vi "Version_2.0_Single_Column_Code.vi"() -> ()   [LabVIEW 2020] (continued)
                          }
                          frame #3 {
                            n8961 = local read "Stopper that ends \nthe main loops"() -> (w9454:bool)
                            n8962 = local read "VISA Refnum in\nfor Pump"() -> (w9455:refnum<visa-resource-name>)
                            n8963 = case shown="True" w9454 {
                              frame False {
                              }
                              frame True {
                                n8964 = local read "VISA Refnum in\nfor Pump"() -> (w9456:refnum<visa-resource-name>)
                                n8965 = call "HardStopCurrentProcess (SubVI).vi"("VISA Refnum in"=w9456) -> ()  [unwired: 11 in]
                              }
                            }
                            n8966 = call "ProcessCompletionWaiter (SubVI).vi"("VISA Refnum in"=w9455) -> ()  [unwired: 11 in]
                          }
                          frame #4 {
                            # "Reads the initial Plunger Position for computing the volume dispensed"
                            n8967 = local read "VISA Refnum in\nfor Pump"() -> (w9458:refnum<visa-resource-name>)
                            n8968 = call "AbsolutePlungerPosition (SubVI).vi"("VISA Refnum in"=w9458) -> ("Plunger Position"=w9457:i32)  [unwired: 10 in]
                            n8969 = local write "Initial Plunger Position"(w9457) -> ()
                          }
                          frame #5 {
                            # "Switch to Port-10"
                            # "Port-10 of the pump is conncted to column-2 of chip"
                            n8970 = local read "VISA Refnum in\nfor Pump"() -> (w9460:refnum<visa-resource-name>)
                            n8971 = call "PortChanger (SubVI).vi"("Port Number"="10", "VISA Refnum in"=w9460) -> ()  [unwired: 10 in]
                          }
                          frame #6 {
                            n8972 = local read "Stopper that ends \nthe main loops"() -> (w9461:bool)
                            n8973 = local read "VISA Refnum in\nfor Pump"() -> (w9462:refnum<visa-resource-name>)
                            n8974 = case shown="True" w9461 {
                              frame False {
                              }
                              frame True {
                                n8975 = local read "VISA Refnum in\nfor Pump"() -> (w9463:refnum<visa-resource-name>)
                                n8976 = call "HardStopCurrentProcess (SubVI).vi"("VISA Refnum in"=w9463) -> ()  [unwired: 11 in]
                              }
                            }
                            n8977 = call "ProcessCompletionWaiter (SubVI).vi"("VISA Refnum in"=w9462) -> ()  [unwired: 11 in]
                          }
                          frame #7 {
                            # "Keeps the AMF valve after column-1 closed and valve after column-2 open"
                            n8978 = local read "Buffer-C2 Dispense\nFlow Rate (ul/min)"() -> (w9476:dbl)
                            n8979 = local read "Buffer-C2 Pumping\nResolution"() -> (w9475:T2)
                            n8980 = local read "VISA Refnum in\nfor Pump"() -> (w9478:refnum<visa-resource-name>)
                            n8981 = local write "Pause Data Collection"(FALSE ("Pause Data Collection")) -> ()
                            n8982 = local write "Valve V1 Open"(FALSE ("Valve V1 Open")) -> ()
                            n8983 = local write "Valve V3 Open"(TRUE ("Valve V3 Open")) -> ()
                            n8984 = local write "Valve V2 Open"(FALSE ("Valve V2 Open")) -> ()
                            n8985 = local write "Valve V4 Open"(TRUE ("Valve V4 Open")) -> ()
                            n8986 = local read "Volume of Syringe"() -> (w9477:dbl)
                            n8987 = call "GoToAbsolutePosition(SubVI).vi"("Absolute Volume Position in Syringe (in ul)"=0.0 ("Volume to be Dispensed"), "Volume of Syringe"=w9477, "Resolution of Pumping"=w9475, "Flow Rate (ul/min)"=w9476, "VISA Refnum in"=w9478) -> ()  [unwired: 6 in, 1 out]
                            n8988 = local write "External Valve \nOpen"(FALSE ("External Valve \nOpen")) -> ()
                            n8989 = local write "Valve V8 Open"(FALSE ("Valve V8 Open")) -> ()
                            n8990 = local write "Valve V7 Open"(TRUE ("Valve V7 Open")) -> ()
                            n8991 = local write "Valve V6 Open"(TRUE ("Valve V6 Open")) -> ()
                            n8992 = local write "Valve V5 Open"(TRUE ("Valve V5 Open")) -> ()
                          }
                          frame #8 {
                            n8993 = local read "Initial Plunger Position"() -> (w9481:dbl)
                            n8994 = local read "Buffer-C2 Pumping\nResolution"() -> (w9480:T2)
                            n8995 = local read "VISA Refnum in\nfor Pump"() -> (w9482:refnum<visa-resource-name>)
                            n8996 = local read "Volume of Syringe"() -> (w9479:dbl)
                            n8997 = while {
                              tunnel: w9481 -> [w9488]
                              tunnel: w9482 -> [w9487]
                              tunnel: w9480 -> [w9486]
                              tunnel: w9479 -> [w9485]
                              stop <- w9483 stop-if-true
                              n8998 = Wait (ms)(milliseconds to wait=u32 100) -> ()  [unwired: 1 out]
                              n8999 = stacked-sequence {
                                tunnel: w9488 -> [w9494 _]
                                tunnel: w9487 -> [w9493 w9514]
                                tunnel: w9486 -> [w9492 _]
                                tunnel: w9485 -> [w9491 _]
                                tunnel: [_ w9511] -> w9483
                                frame #0 {
                                n9000 = call "AbsolutePlungerPosition (SubVI).vi"("VISA Refnum in"=w9493) -> ("Plunger Position"=w9490:i32)  [unwired: 10 in]
                                n9001 = case shown="\"Standard Pumping\", Default" w9492 {
                                tunnel: w9494 -> [w9499 w9508]
                                tunnel: w9490 -> [w9500 w9507]
                                tunnel: [w9498 w9505] -> w9489
                                tunnel: w9491 -> [w9497 w9506]
                                frame "Standard Pumping", Default {
                                n9002 = Subtract(x=w9499, y=w9500) -> (x-y=w9496:dbl)
                                n9003 = Absolute Value(x=w9496) -> (abs(x)=w9495:dbl)
                                n9004 = Multiply(x=w9495, y=w9497) -> (x*y=w9502:dbl)
                                n9005 = Divide(x=w9502, y=3000.0) -> (x/y=w9498:dbl)
                                }
                                frame "High Resolution Pumping" {
                                n9006 = Subtract(x=w9508, y=w9507) -> (x-y=w9504:dbl)
                                n9007 = Absolute Value(x=w9504) -> (abs(x)=w9503:dbl)
                                n9008 = Multiply(x=w9503, y=w9506) -> (x*y=w9510:dbl)
                                n9009 = Divide(x=w9510, y=24000.0) -> (x/y=w9505:dbl)
                                }
                                }
                                n9010 = local write "Volume being Injected \nin this process"(w9489) -> ()
                                }
                                frame #1 {
                                n9011 = call "LSPOneStatus (SubVI).vi"("VISA Refnum in"=w9514) -> ("read buffer"=w9516:string)  [unwired: 10 in]
                                n9012 = local read "Stopper that ends \nthe main loops"() -> (w9513:bool)
                                n9013 = call <vilib>:"Trim Whitespace.vi"("string"=w9516) -> ("trimmed string"=w9515:string)  [unwired: 1 in]
                                n9014 = Equal?(x=w9515, y="/0`\u0003") -> (x = y?=w9512:bool)
                                n9015 = Or(x=w9512, y=w9513) -> (x .or. y?=w9511:bool)
                                }
                              }
                            }
                          }
                          frame #9 {
                            n9016 = local read "Stop for End of \nExperiment \nand Data Writing"() -> (w9518:bool)
                            n9017 = local write "Pause Data Collection"(TRUE ("Pause Data Collection")) -> ()
                            n9018 = local write "Valve V2 Open"(FALSE ("Valve V2 Open")) -> ()
                            n9019 = local write "Valve V1 Open"(FALSE ("Valve V1 Open")) -> ()
                            n9020 = local write "Valve V3 Open"(FALSE ("Valve V3 Open")) -> ()
                            n9021 = local write "Valve V4 Open"(FALSE ("Valve V4 Open")) -> ()
                            n9022 = local write "Start the Process"(FALSE) -> ()
                            n9023 = Wait (ms)(milliseconds to wait=u32 500) -> ()  [unwired: 1 out]
                            n9024 = case shown="True" w9518 {
                              frame False {
                              }
                              frame True {
                                n9025 = local read "VISA Refnum in\nfor Pump"() -> (w9531:refnum<visa-resource-name>)
                                n9026 = call "HardStopCurrentProcess (SubVI).vi"("VISA Refnum in"=w9531) -> ()  [unwired: 11 in]
                              }
                            }
                            n9027 = local write "External Valve \nOpen"(FALSE ("External Valve \nOpen")) -> ()
                            n9028 = local write "Valve V8 Open"(FALSE ("Valve V8 Open")) -> ()
                            n9029 = local write "Valve V6 Open"(FALSE ("Valve V6 Open")) -> ()
                            n9030 = local write "Valve V5 Open"(FALSE ("Valve V5 Open")) -> ()
                            n9031 = local write "Valve V7 Open"(FALSE ("Valve V7 Open")) -> ()
                          }
                          frame #10 {
                            n9032 = local write "Volume being Injected \nin this process"(0.0 ("Volume being Injected \nin this process")) -> ()
                          }
                        }
                      }
                    }
                  }
                }
              }
              frame True {
                n9033 = local write "Pause Data Collection"(FALSE ("Pause Data Collection")) -> ()
              }
            }
          }
          frame "Initialize Only the Valve" {
            n9034 = local read "Stop for End of \nExperiment \nand Data Writing"() -> (w9534:bool)
            n9035 = case shown="False" w9534 {
              frame False {
                n9036 = local read "Start the Process"() -> (w9535:bool)
                n9037 = case shown="True" w9535 {
                  frame False {
                    n9038 = local read "Stopper that ends \nthe main loops"() -> (w9537:bool)
                    n9039 = local read "Start the Process"() -> (w9538:bool)
                    n9040 = Or(x=w9538, y=w9537) -> (x .or. y?=w9536:bool)
                    n9041 = case shown="False" w9536 {
                      frame False {
                        n9042 = while {
                          stop <- w9541 stop-if-true
                          n9043 = local read "Stopper that ends \nthe main loops"() -> (w9543:bool)
                          n9044 = local read "Start the Process"() -> (w9542:bool)
                          n9045 = Or(x=w9542, y=w9543) -> (x .or. y?=w9541:bool)
                          n9046 = Wait (ms)(milliseconds to wait=u32 10) -> ()  [unwired: 1 out]
                        }
                        n9047 = One Button Dialog(message="Please select the process and press the 'Start Process' Button") -> ()  [unwired: 1 in, 1 out]
                      }
                      frame True {
                      }
                    }
                  }
                  frame True {
                    n9048 = stacked-sequence {
                      frame #0 {
                        n9049 = local read "VISA Refnum in\nfor Valve"() -> (w9544:refnum<visa-resource-name>)
                        n9050 = call "Initializer_Valve (SubVI).vi"("VISA Refnum in"=w9544) -> ()  [unwired: 11 in]
                      }
                      frame #1 {
                        n9051 = local read "VISA Refnum in\nfor Valve"() -> (w9545:refnum<visa-resource-name>)
                        n9052 = call "ProcessCompletionWaiter (SubVI).vi"("VISA Refnum in"=w9545) -> ()  [unwired: 11 in]
                      }
                      frame #2 {
                        n9053 = local write "Start the Process"(FALSE ("Start the Process")) -> ()
                      }
                    }
                  }
                }
              }
              frame True {
              }
            }
          }
          frame "Clean the tubing from Ports 3,4,5 and 7" {
            n9054 = local read "Stopper that ends \nthe main loops"() -> (w9547:bool)
            n9055 = case shown="False" w9547 {
              frame False {
                n9056 = local read "Start the Process"() -> (w9548:bool)
                n9057 = case shown="True" w9548 {
                  frame False {
                    n9058 = local read "Stopper that ends \nthe main loops"() -> (w9550:bool)
                    n9059 = local read "Start the Process"() -> (w9549:bool)
                    n9060 = Or(x=w9550, y=w9549) -> (x .or. y?=w9551:bool)
                    n9061 = case shown="False" w9551 {
                      frame False {
                        n9062 = while {
                          stop <- w9554 stop-if-true
                          n9063 = local read "Stopper that ends \nthe main loops"() -> (w9556:bool)
                          n9064 = local read "Stop for End of \nExperiment \nand Data Writing"() -> (w9553:bool)
                          n9065 = local read "Start the Process"() -> (w9555:bool)
                          n9066 = Wait (ms)(milliseconds to wait=u32 10) -> ()  [unwired: 1 out]
                          n9067 = Or(x=w9556, y=w9555) -> (x .or. y?=w9554:bool)
                          n9068 = local write "Stopper that ends \nthe main loops"(w9553) -> ()
                        }
                        n9069 = One Button Dialog(message="Please Select the Process and Press 'Start the Process' Button") -> ()  [unwired: 1 in, 1 out]
                      }
                      frame True {
                      }
                    }
                  }
                  frame True {
                    n9070 = stacked-sequence {
                      frame #0 {
                        n9071 = for {
                          N: 2 -> [_]
                          n9072 = stacked-sequence {
                            frame #0 {
                              # "Switch to Port-4"
                              # "Port-4 of pump is connected to Buffer-A"
                              n9073 = local read "VISA Refnum in\nfor Pump"() -> (w9561:refnum<visa-resource-name>)
                              n9074 = local write "Pause Data Collection"(TRUE ("Pause Data Collection")) -> ()
                              n9075 = call "PortChanger (SubVI).vi"("Port Number"="3", "VISA Refnum in"=w9561) -> ()  [unwired: 10 in]
                            }
                            frame #1 {
                              n9076 = local read "VISA Refnum in\nfor Pump"() -> (w9562:refnum<visa-resource-name>)
                              n9077 = call "ProcessCompletionWaiter (SubVI).vi"("VISA Refnum in"=w9562) -> ()  [unwired: 11 in]
                            }
                            frame #2 {
                              n9078 = local read "VISA Refnum in\nfor Pump"() -> (w9567:refnum<visa-resource-name>)
                              n9079 = local read "Volume of Syringe"() -> (w9566:dbl)
                              n9080 = call "RPickUp(SubVI).vi"("Volume to be picked up"=10.0, "Volume of Syringe"=w9566, "Resolution of PickUP"=T2."Standard Pumping", "PickUp Flow Rate (ul/min)"=15.0, "VISA Refnum in"=w9567) -> ()  [unwired: 6 in, 1 out]
                            }
                            frame #3 {
                              n9081 = local read "Stopper that ends \nthe main loops"() -> (w9568:bool)
                              n9082 = local read "VISA Refnum in\nfor Pump"() -> (w9569:refnum<visa-resource-name>)
                              n9083 = case shown="True" w9568 {
                                frame False {
                                }
                                frame True {
                                n9084 = local read "VISA Refnum in\nfor Pump"() -> (w9570:refnum<visa-resource-name>)
                                n9085 = call "HardStopCurrentProcess (SubVI).vi"("VISA Refnum in"=w9570) -> ()  [unwired: 11 in]
                                }
                              }
                              n9086 = call "ProcessCompletionWaiter (SubVI).vi"("VISA Refnum in"=w9569) -> ()  [unwired: 11 in]
                            }
                            frame #4 {
                              # "Switch to Port-1"
                              # "Port-1 of the pump is conncted to Waste"
                              n9087 = local read "VISA Refnum in\nfor Pump"() -> (w9572:refnum<visa-resource-name>)
                              n9088 = call "PortChanger (SubVI).vi"("Port Number"="1", "VISA Refnum in"=w9572) -> ()  [unwired: 10 in]
                            }
                            frame #5 {
                              n9089 = local read "Stopper that ends \nthe main loops"() -> (w9573:bool)
                              n9090 = local read "VISA Refnum in\nfor Pump"() -> (w9574:refnum<visa-resource-name>)
                              n9091 = case shown="True" w9573 {
                                frame False {
                                }
                                frame True {
                                n9092 = local read "VISA Refnum in\nfor Pump"() -> (w9575:refnum<visa-resource-name>)
                                n9093 = call "HardStopCurrentProcess (SubVI).vi"("VISA Refnum in"=w9575) -> ()  [unwired: 11 in]
                                }
                              }
                              n9094 = call "ProcessCompletionWaiter (SubVI).vi"("VISA Refnum in"=w9574) -> ()  [unwired: 11 in]
                            }
                            frame #6 {
                              n9095 = local read "VISA Refnum in\nfor Pump"() -> (w9580:refnum<visa-resource-name>)
                              n9096 = local read "Volume of Syringe"() -> (w9579:dbl)
                              n9097 = call "GoToAbsolutePosition(SubVI).vi"("Absolute Volume Position in Syringe (in ul)"=0.0 ("Volume to be Dispensed"), "Volume of Syringe"=w9579, "Resolution of Pumping"=T2."Standard Pumping" ("Resolution for Dispensing"), "Flow Rate (ul/min)"=150.0 ("Dispense Flow Rate (ul/min)"), "VISA Refnum in"=w9580) -> ()  [unwired: 6 in, 1 out]
                            }
                            frame #7 {
                              n9098 = local read "Stopper that ends \nthe main loops"() -> (w9582:bool)
                              n9099 = case shown="True" w9582 {
                                frame False {
                                }
                                frame True {
                                n9100 = local read "VISA Refnum in\nfor Pump"() -> (w9583:refnum<visa-resource-name>)
                                n9101 = call "HardStopCurrentProcess (SubVI).vi"("VISA Refnum in"=w9583) -> ()  [unwired: 11 in]
                                }
                              }
                              n9102 = local read "VISA Refnum in\nfor Pump"() -> (w9581:refnum<visa-resource-name>)
                              n9103 = call "ProcessCompletionWaiter (SubVI).vi"("VISA Refnum in"=w9581) -> ()  [unwired: 11 in]
                            }
                          }
                        }
                      }
                      frame #1 {
                        n9104 = local read "No. of \ncleaning cycles"() -> (w9584:i32)
                        n9105 = for {
                          N: w9584 -> [_]
                          n9106 = stacked-sequence {
                            frame #0 {
                              # "Switch to Port-4"
                              # "Port-4 of pump is connected to Buffer-A"
                              n9107 = local read "VISA Refnum in\nfor Pump"() -> (w9587:refnum<visa-resource-name>)
                              n9108 = local write "Pause Data Collection"(TRUE ("Pause Data Collection")) -> ()
                              n9109 = call "PortChanger (SubVI).vi"("Port Number"="4", "VISA Refnum in"=w9587) -> ()  [unwired: 10 in]
                            }
                            frame #1 {
                              n9110 = local read "VISA Refnum in\nfor Pump"() -> (w9588:refnum<visa-resource-name>)
                              n9111 = call "ProcessCompletionWaiter (SubVI).vi"("VISA Refnum in"=w9588) -> ()  [unwired: 11 in]
                            }
                            frame #2 {
                              n9112 = local read "VISA Refnum in\nfor Pump"() -> (w9593:refnum<visa-resource-name>)
                              n9113 = local read "Apparent Volume\nof Syringe"() -> (w9589:dbl)
                              n9114 = local read "Volume of Syringe"() -> (w9592:dbl)
                              n9115 = call "RPickUp(SubVI).vi"("Volume to be picked up"=w9589, "Volume of Syringe"=w9592, "Resolution of PickUP"=T2."Standard Pumping", "PickUp Flow Rate (ul/min)"=150.0, "VISA Refnum in"=w9593) -> ()  [unwired: 6 in, 1 out]
                            }
                            frame #3 {
                              n9116 = local read "Stopper that ends \nthe main loops"() -> (w9594:bool)
                              n9117 = local read "VISA Refnum in\nfor Pump"() -> (w9595:refnum<visa-resource-name>)
                              n9118 = case shown="True" w9594 {
                                frame False {
                                }
                                frame True {
                                n9119 = local read "VISA Refnum in\nfor Pump"() -> (w9596:refnum<visa-resource-name>)
                                n9120 = call "HardStopCurrentProcess (SubVI).vi"("VISA Refnum in"=w9596) -> ()  [unwired: 11 in]
                                }
                              }
                              n9121 = call "ProcessCompletionWaiter (SubVI).vi"("VISA Refnum in"=w9595) -> ()  [unwired: 11 in]
                            }
                            frame #4 {
                              # "Switch to Port-1"
                              # "Port-1 of the pump is conncted to Waste"
                              n9122 = local read "VISA Refnum in\nfor Pump"() -> (w9598:refnum<visa-resource-name>)
                              n9123 = call "PortChanger (SubVI).vi"("Port Number"="1", "VISA Refnum in"=w9598) -> ()  [unwired: 10 in]
                            }
                            frame #5 {
                              n9124 = local read "Stopper that ends \nthe main loops"() -> (w9599:bool)
                              n9125 = local read "VISA Refnum in\nfor Pump"() -> (w9600:refnum<visa-resource-name>)
                              n9126 = case shown="True" w9599 {
                                frame False {
                                }
                                frame True {
                                n9127 = local read "VISA Refnum in\nfor Pump"() -> (w9601:refnum<visa-resource-name>)
                                n9128 = call "HardStopCurrentProcess (SubVI).vi"("VISA Refnum in"=w9601) -> ()  [unwired: 11 in]
                                }
                              }
                              n9129 = call "ProcessCompletionWaiter (SubVI).vi"("VISA Refnum in"=w9600) -> ()  [unwired: 11 in]
                            }
                            frame #6 {
                              n9130 = local read "VISA Refnum in\nfor Pump"() -> (w9606:refnum<visa-resource-name>)
                              n9131 = local read "Volume of Syringe"() -> (w9605:dbl)
                              n9132 = call "GoToAbsolutePosition(SubVI).vi"("Absolute Volume Position in Syringe (in ul)"=0.0 ("Volume to be Dispensed"), "Volume of Syringe"=w9605, "Resolution of Pumping"=T2."Standard Pumping" ("Resolution for Dispensing"), "Flow Rate (ul/min)"=150.0 ("Dispense Flow Rate (ul/min)"), "VISA Refnum in"=w9606) -> ()  [unwired: 6 in, 1 out]
                            }
                            frame #7 {
                              n9133 = local read "Stopper that ends \nthe main loops"() -> (w9608:bool)
                              n9134 = case shown="True" w9608 {
                                frame False {
                                }
                                frame True {
                                n9135 = local read "VISA Refnum in\nfor Pump"() -> (w9609:refnum<visa-resource-name>)
                                n9136 = call "HardStopCurrentProcess (SubVI).vi"("VISA Refnum in"=w9609) -> ()  [unwired: 11 in]
                                }
                              }
                              n9137 = local read "VISA Refnum in\nfor Pump"() -> (w9607:refnum<visa-resource-name>)
                              n9138 = call "ProcessCompletionWaiter (SubVI).vi"("VISA Refnum in"=w9607) -> ()  [unwired: 11 in]
                            }
                          }
                        }
                      }
                      frame #2 {
                        n9139 = local read "No. of \ncleaning cycles"() -> (w9610:i32)
                        n9140 = for {
                          N: w9610 -> [_]
                          n9141 = stacked-sequence {
                            frame #0 {
                              # "Switch to Port-4"
                              # "Port-4 of pump is connected to Buffer-A"
                              n9142 = local read "VISA Refnum in\nfor Pump"() -> (w9613:refnum<visa-resource-name>)
                              n9143 = local write "Pause Data Collection"(TRUE ("Pause Data Collection")) -> ()
                              n9144 = call "PortChanger (SubVI).vi"("Port Number"="5", "VISA Refnum in"=w9613) -> ()  [unwired: 10 in]
                            }
                            frame #1 {
                              n9145 = local read "VISA Refnum in\nfor Pump"() -> (w9614:refnum<visa-resource-name>)
                              n9146 = call "ProcessCompletionWaiter (SubVI).vi"("VISA Refnum in"=w9614) -> ()  [unwired: 11 in]
                            }
                            frame #2 {
                              n9147 = local read "VISA Refnum in\nfor Pump"() -> (w9619:refnum<visa-resource-name>)
                              n9148 = local read "Apparent Volume\nof Syringe"() -> (w9615:dbl)
                              n9149 = local read "Volume of Syringe"() -> (w9618:dbl)
                              n9150 = call "RPickUp(SubVI).vi"("Volume to be picked up"=w9615, "Volume of Syringe"=w9618, "Resolution of PickUP"=T2."Standard Pumping", "PickUp Flow Rate (ul/min)"=150.0, "VISA Refnum in"=w9619) -> ()  [unwired: 6 in, 1 out]
                            }
                            frame #3 {
                              n9151 = local read "Stopper that ends \nthe main loops"() -> (w9620:bool)
                              n9152 = local read "VISA Refnum in\nfor Pump"() -> (w9621:refnum<visa-resource-name>)
                              n9153 = case shown="True" w9620 {
                                frame False {
                                }
                                frame True {
                                n9154 = local read "VISA Refnum in\nfor Pump"() -> (w9622:refnum<visa-resource-name>)
                                n9155 = call "HardStopCurrentProcess (SubVI).vi"("VISA Refnum in"=w9622) -> ()  [unwired: 11 in]
                                }
                              }
                              n9156 = call "ProcessCompletionWaiter (SubVI).vi"("VISA Refnum in"=w9621) -> ()  [unwired: 11 in]
                            }
                            frame #4 {
                              # "Switch to Port-1"
                              # "Port-1 of the pump is conncted to Waste"
                              n9157 = local read "VISA Refnum in\nfor Pump"() -> (w9624:refnum<visa-resource-name>)
                              n9158 = call "PortChanger (SubVI).vi"("Port Number"="1", "VISA Refnum in"=w9624) -> ()  [unwired: 10 in]
                            }
                            frame #5 {
                              n9159 = local read "Stopper that ends \nthe main loops"() -> (w9625:bool)
                              n9160 = local read "VISA Refnum in\nfor Pump"() -> (w9626:refnum<visa-resource-name>)
                              n9161 = case shown="True" w9625 {
                                frame False {
                                }
                                frame True {
                                n9162 = local read "VISA Refnum in\nfor Pump"() -> (w9627:refnum<visa-resource-name>)
                                n9163 = call "HardStopCurrentProcess (SubVI).vi"("VISA Refnum in"=w9627) -> ()  [unwired: 11 in]
                                }
                              }
                              n9164 = call "ProcessCompletionWaiter (SubVI).vi"("VISA Refnum in"=w9626) -> ()  [unwired: 11 in]
                            }
                            frame #6 {
                              n9165 = local read "VISA Refnum in\nfor Pump"() -> (w9632:refnum<visa-resource-name>)
                              n9166 = local read "Volume of Syringe"() -> (w9631:dbl)
                              n9167 = call "GoToAbsolutePosition(SubVI).vi"("Absolute Volume Position in Syringe (in ul)"=0.0 ("Volume to be Dispensed"), "Volume of Syringe"=w9631, "Resolution of Pumping"=T2."Standard Pumping" ("Resolution for Dispensing"), "Flow Rate (ul/min)"=150.0 ("Dispense Flow Rate (ul/min)"), "VISA Refnum in"=w9632) -> ()  [unwired: 6 in, 1 out]
                            }
                            frame #7 {
                              n9168 = local read "Stopper that ends \nthe main loops"() -> (w9634:bool)
                              n9169 = case shown="True" w9634 {
                                frame False {
                                }
                                frame True {
                                n9170 = local read "VISA Refnum in\nfor Pump"() -> (w9635:refnum<visa-resource-name>)
                                n9171 = call "HardStopCurrentProcess (SubVI).vi"("VISA Refnum in"=w9635) -> ()  [unwired: 11 in]
                                }
                              }
                              n9172 = local read "VISA Refnum in\nfor Pump"() -> (w9633:refnum<visa-resource-name>)
                              n9173 = call "ProcessCompletionWaiter (SubVI).vi"("VISA Refnum in"=w9633) -> ()  [unwired: 11 in]
                            }
                          }
                        }
                      }
                      frame #3 {
                        n9174 = local read "No. of \ncleaning cycles"() -> (w9636:i32)
                        n9175 = for {
                          N: w9636 -> [_]
                          n9176 = stacked-sequence {
                            frame #0 {
                              # "Switch to Port-4"
                              # "Port-4 of pump is connected to Buffer-A"
                              n9177 = local read "VISA Refnum in\nfor Pump"() -> (w9639:refnum<visa-resource-name>)
                              n9178 = local write "Pause Data Collection"(TRUE ("Pause Data Collection")) -> ()
                              n9179 = call "PortChanger (SubVI).vi"("Port Number"="7", "VISA Refnum in"=w9639) -> ()  [unwired: 10 in]
                            }
                            frame #1 {
                              n9180 = local read "VISA Refnum in\nfor Pump"() -> (w9640:refnum<visa-resource-name>)
                              n9181 = call "ProcessCompletionWaiter (SubVI).vi"("VISA Refnum in"=w9640) -> ()  [unwired: 11 in]
                            }
                            frame #2 {
                              n9182 = local read "VISA Refnum in\nfor Pump"() -> (w9645:refnum<visa-resource-name>)
                              n9183 = local read "Apparent Volume\nof Syringe"() -> (w9641:dbl)
                              n9184 = local read "Volume of Syringe"() -> (w9644:dbl)
                              n9185 = call "RPickUp(SubVI).vi"("Volume to be picked up"=w9641, "Volume of Syringe"=w9644, "Resolution of PickUP"=T2."Standard Pumping", "PickUp Flow Rate (ul/min)"=150.0, "VISA Refnum in"=w9645) -> ()  [unwired: 6 in, 1 out]
                            }
                            frame #3 {
                              n9186 = local read "Stopper that ends \nthe main loops"() -> (w9646:bool)
                              n9187 = local read "VISA Refnum in\nfor Pump"() -> (w9647:refnum<visa-resource-name>)
                              n9188 = case shown="True" w9646 {
                                frame False {
                                }
                                frame True {
                                n9189 = local read "VISA Refnum in\nfor Pump"() -> (w9648:refnum<visa-resource-name>)
                                n9190 = call "HardStopCurrentProcess (SubVI).vi"("VISA Refnum in"=w9648) -> ()  [unwired: 11 in]
                                }
                              }
                              n9191 = call "ProcessCompletionWaiter (SubVI).vi"("VISA Refnum in"=w9647) -> ()  [unwired: 11 in]
                            }
                            frame #4 {
                              # "Switch to Port-1"
                              # "Port-1 of the pump is conncted to Waste"
                              n9192 = local read "VISA Refnum in\nfor Pump"() -> (w9650:refnum<visa-resource-name>)
                              n9193 = call "PortChanger (SubVI).vi"("Port Number"="1", "VISA Refnum in"=w9650) -> ()  [unwired: 10 in]
                            }
                            frame #5 {
                              n9194 = local read "Stopper that ends \nthe main loops"() -> (w9651:bool)
                              n9195 = local read "VISA Refnum in\nfor Pump"() -> (w9652:refnum<visa-resource-name>)
                              n9196 = case shown="True" w9651 {
                                frame False {
                                }
                                frame True {
                                n9197 = local read "VISA Refnum in\nfor Pump"() -> (w9653:refnum<visa-resource-name>)
                                n9198 = call "HardStopCurrentProcess (SubVI).vi"("VISA Refnum in"=w9653) -> ()  [unwired: 11 in]
                                }
                              }
                              n9199 = call "ProcessCompletionWaiter (SubVI).vi"("VISA Refnum in"=w9652) -> ()  [unwired: 11 in]
                            }
                            frame #6 {
                              n9200 = local read "VISA Refnum in\nfor Pump"() -> (w9658:refnum<visa-resource-name>)
                              n9201 = local read "Volume of Syringe"() -> (w9657:dbl)
                              n9202 = call "GoToAbsolutePosition(SubVI).vi"("Absolute Volume Position in Syringe (in ul)"=0.0 ("Volume to be Dispensed"), "Volume of Syringe"=w9657, "Resolution of Pumping"=T2."Standard Pumping" ("Resolution for Dispensing"), "Flow Rate (ul/min)"=150.0 ("Dispense Flow Rate (ul/min)"), "VISA Refnum in"=w9658) -> ()  [unwired: 6 in, 1 out]
                            }
                            frame #7 {
                              n9203 = local read "Stopper that ends \nthe main loops"() -> (w9660:bool)
                              n9204 = case shown="True" w9660 {
                                frame False {
                                }
                                frame True {
                                n9205 = local read "VISA Refnum in\nfor Pump"() -> (w9661:refnum<visa-resource-name>)
                                n9206 = call "HardStopCurrentProcess (SubVI).vi"("VISA Refnum in"=w9661) -> ()  [unwired: 11 in]
                                }
                              }
                              n9207 = local read "VISA Refnum in\nfor Pump"() -> (w9659:refnum<visa-resource-name>)
                              n9208 = call "ProcessCompletionWaiter (SubVI).vi"("VISA Refnum in"=w9659) -> ()  [unwired: 11 in]
                            }
                          }
                        }
                      }
                      frame #4 {
                        n9209 = local write "Start the Process"(FALSE ("Start the Process")) -> ()
                      }
                    }
                  }
                }
              }
              frame True {
                n9210 = local write "Pause Data Collection"(FALSE ("Pause Data Collection")) -> ()
              }
            }
          }
          frame "Clean the tubing from Ports 3,4,7 and wash the column" {
            n9211 = local read "Stopper that ends \nthe main loops"() -> (w9664:bool)
            n9212 = case shown="False" w9664 {
              frame False {
                n9213 = local read "Start the Process"() -> (w9665:bool)
                n9214 = case shown="True" w9665 {
                  frame False {
                    n9215 = local read "Stopper that ends \nthe main loops"() -> (w9667:bool)
                    n9216 = local read "Start the Process"() -> (w9666:bool)
                    n9217 = Or(x=w9667, y=w9666) -> (x .or. y?=w9668:bool)
                    n9218 = case shown="False" w9668 {
                      frame False {
                        n9219 = while {
                          stop <- w9671 stop-if-true
                          n9220 = local read "Stopper that ends \nthe main loops"() -> (w9673:bool)
                          n9221 = local read "Stop for End of \nExperiment \nand Data Writing"() -> (w9670:bool)
                          n9222 = local read "Start the Process"() -> (w9672:bool)
                          n9223 = Wait (ms)(milliseconds to wait=u32 10) -> ()  [unwired: 1 out]
                          n9224 = Or(x=w9673, y=w9672) -> (x .or. y?=w9671:bool)
                          n9225 = local write "Stopper that ends \nthe main loops"(w9670) -> ()
                        }
                        n9226 = One Button Dialog(message="Please Select the Process and Press 'Start the Process' Button") -> ()  [unwired: 1 in, 1 out]
                      }
                      frame True {
                      }
                    }
                  }
                  frame True {
                    n9227 = stacked-sequence {
                      frame #0 {
                        n9228 = for {
                          N: 2 -> [_]
                          n9229 = stacked-sequence {
                            frame #0 {
                              # "Switch to Port-4"
                              # "Port-4 of pump is connected to Buffer-A"
                              n9230 = local read "VISA Refnum in\nfor Pump"() -> (w9678:refnum<visa-resource-name>)
                              n9231 = local write "Pause Data Collection"(TRUE ("Pause Data Collection")) -> ()
                              n9232 = call "PortChanger (SubVI).vi"("Port Number"="3", "VISA Refnum in"=w9678) -> ()  [unwired: 10 in]
                            }
                            frame #1 {
                              n9233 = local read "VISA Refnum in\nfor Pump"() -> (w9679:refnum<visa-resource-name>)
                              n9234 = call "ProcessCompletionWaiter (SubVI).vi"("VISA Refnum in"=w9679) -> ()  [unwired: 11 in]
                            }
                            frame #2 {
                              n9235 = local read "VISA Refnum in\nfor Pump"() -> (w9684:refnum<visa-resource-name>)
                              n9236 = local read "Volume of Syringe"() -> (w9683:dbl)
                              n9237 = call "RPickUp(SubVI).vi"("Volume to be picked up"=10.0, "Volume of Syringe"=w9683, "Resolution of PickUP"=T2."Standard Pumping", "PickUp Flow Rate (ul/min)"=15.0, "VISA Refnum in"=w9684) -> ()  [unwired: 6 in, 1 out]
                            }
                            frame #3 {
                              n9238 = local read "Stopper that ends \nthe main loops"() -> (w9685:bool)
                              n9239 = local read "VISA Refnum in\nfor Pump"() -> (w9686:refnum<visa-resource-name>)
                              n9240 = case shown="True" w9685 {
                                frame False {
                                }
                                frame True {
                                n9241 = local read "VISA Refnum in\nfor Pump"() -> (w9687:refnum<visa-resource-name>)
                                n9242 = call "HardStopCurrentProcess (SubVI).vi"("VISA Refnum in"=w9687) -> ()  [unwired: 11 in]
                                }
                              }
                              n9243 = call "ProcessCompletionWaiter (SubVI).vi"("VISA Refnum in"=w9686) -> ()  [unwired: 11 in]
                            }
                            frame #4 {
                              # "Switch to Port-1"
                              # "Port-1 of the pump is conncted to Waste"
                              n9244 = local read "VISA Refnum in\nfor Pump"() -> (w9689:refnum<visa-resource-name>)
                              n9245 = call "PortChanger (SubVI).vi"("Port Number"="1", "VISA Refnum in"=w9689) -> ()  [unwired: 10 in]
                            }
                            frame #5 {
                              n9246 = local read "Stopper that ends \nthe main loops"() -> (w9690:bool)
                              n9247 = local read "VISA Refnum in\nfor Pump"() -> (w9691:refnum<visa-resource-name>)
                              n9248 = case shown="True" w9690 {
                                frame False {
                                }
                                frame True {
                                n9249 = local read "VISA Refnum in\nfor Pump"() -> (w9692:refnum<visa-resource-name>)
                                n9250 = call "HardStopCurrentProcess (SubVI).vi"("VISA Refnum in"=w9692) -> ()  [unwired: 11 in]
                                }
                              }
                              n9251 = call "ProcessCompletionWaiter (SubVI).vi"("VISA Refnum in"=w9691) -> ()  [unwired: 11 in]
                            }
                            frame #6 {
                              n9252 = local read "VISA Refnum in\nfor Pump"() -> (w9697:refnum<visa-resource-name>)
                              n9253 = local read "Volume of Syringe"() -> (w9696:dbl)
                              n9254 = call "GoToAbsolutePosition(SubVI).vi"("Absolute Volume Position in Syringe (in ul)"=0.0 ("Volume to be Dispensed"), "Volume of Syringe"=w9696, "Resolution of Pumping"=T2."Standard Pumping" ("Resolution for Dispensing"), "Flow Rate (ul/min)"=150.0 ("Dispense Flow Rate (ul/min)"), "VISA Refnum in"=w9697) -> ()  [unwired: 6 in, 1 out]
                            }
                            frame #7 {
                              n9255 = local read "Stopper that ends \nthe main loops"() -> (w9699:bool)
                              n9256 = case shown="True" w9699 {
                                frame False {
                                }
                                frame True {
                                n9257 = local read "VISA Refnum in\nfor Pump"() -> (w9700:refnum<visa-resource-name>)
                                n9258 = call "HardStopCurrentProcess (SubVI).vi"("VISA Refnum in"=w9700) -> ()  [unwired: 11 in]
                                }
                              }
                              n9259 = local read "VISA Refnum in\nfor Pump"() -> (w9698:refnum<visa-resource-name>)
                              n9260 = call "ProcessCompletionWaiter (SubVI).vi"("VISA Refnum in"=w9698) -> ()  [unwired: 11 in]
                            }
                          }
                        }
                      }
                      frame #1 {
                        n9261 = local read "No. of \ncleaning cycles"() -> (w9701:i32)
                        n9262 = for {
                          N: w9701 -> [_]
                          n9263 = stacked-sequence {
                            frame #0 {
                              # "Switch to Port-4"
                              # "Port-4 of pump is connected to Buffer-A"
                              n9264 = local read "VISA Refnum in\nfor Pump"() -> (w9704:refnum<visa-resource-name>)
                              n9265 = local write "Pause Data Collection"(TRUE ("Pause Data Collection")) -> ()
                              n9266 = call "PortChanger (SubVI).vi"("Port Number"="4", "VISA Refnum in"=w9704) -> ()  [unwired: 10 in]
                            }
                            frame #1 {
                              n9267 = local read "VISA Refnum in\nfor Pump"() -> (w9705:refnum<visa-resource-name>)
                              n9268 = call "ProcessCompletionWaiter (SubVI).vi"("VISA Refnum in"=w9705) -> ()  [unwired: 11 in]
                            }
                            frame #2 {
                              n9269 = local read "VISA Refnum in\nfor Pump"() -> (w9710:refnum<visa-resource-name>)
                              n9270 = local read "Apparent Volume\nof Syringe"() -> (w9706:dbl)
                              n9271 = local read "Volume of Syringe"() -> (w9709:dbl)
                              n9272 = call "RPickUp(SubVI).vi"("Volume to be picked up"=w9706, "Volume of Syringe"=w9709, "Resolution of PickUP"=T2."Standard Pumping", "PickUp Flow Rate (ul/min)"=150.0, "VISA Refnum in"=w9710) -> ()  [unwired: 6 in, 1 out]
                            }
                            frame #3 {
                              n9273 = local read "Stopper that ends \nthe main loops"() -> (w9711:bool)
                              n9274 = local read "VISA Refnum in\nfor Pump"() -> (w9712:refnum<visa-resource-name>)
                              n9275 = case shown="True" w9711 {
                                frame False {
                                }
                                frame True {
                                n9276 = local read "VISA Refnum in\nfor Pump"() -> (w9713:refnum<visa-resource-name>)
                                n9277 = call "HardStopCurrentProcess (SubVI).vi"("VISA Refnum in"=w9713) -> ()  [unwired: 11 in]
                                }
                              }
                              n9278 = call "ProcessCompletionWaiter (SubVI).vi"("VISA Refnum in"=w9712) -> ()  [unwired: 11 in]
                            }
                            frame #4 {
                              # "Switch to Port-1"
                              # "Port-1 of the pump is conncted to Waste"
                              n9279 = local read "VISA Refnum in\nfor Pump"() -> (w9715:refnum<visa-resource-name>)
                              n9280 = call "PortChanger (SubVI).vi"("Port Number"="1", "VISA Refnum in"=w9715) -> ()  [unwired: 10 in]
                            }
                            frame #5 {
                              n9281 = local read "Stopper that ends \nthe main loops"() -> (w9716:bool)
                              n9282 = local read "VISA Refnum in\nfor Pump"() -> (w9717:refnum<visa-resource-name>)
                              n9283 = case shown="True" w9716 {
                                frame False {
                                }
                                frame True {
                                n9284 = local read "VISA Refnum in\nfor Pump"() -> (w9718:refnum<visa-resource-name>)
                                n9285 = call "HardStopCurrentProcess (SubVI).vi"("VISA Refnum in"=w9718) -> ()  [unwired: 11 in]
                                }
                              }
                              n9286 = call "ProcessCompletionWaiter (SubVI).vi"("VISA Refnum in"=w9717) -> ()  [unwired: 11 in]
                            }
                            frame #6 {
                              n9287 = local read "VISA Refnum in\nfor Pump"() -> (w9723:refnum<visa-resource-name>)
                              n9288 = local read "Volume of Syringe"() -> (w9722:dbl)
                              n9289 = call "GoToAbsolutePosition(SubVI).vi"("Absolute Volume Position in Syringe (in ul)"=0.0 ("Volume to be Dispensed"), "Volume of Syringe"=w9722, "Resolution of Pumping"=T2."Standard Pumping" ("Resolution for Dispensing"), "Flow Rate (ul/min)"=150.0 ("Dispense Flow Rate (ul/min)"), "VISA Refnum in"=w9723) -> ()  [unwired: 6 in, 1 out]
                            }
                            frame #7 {
                              n9290 = local read "Stopper that ends \nthe main loops"() -> (w9725:bool)
                              n9291 = case shown="True" w9725 {
                                frame False {
                                }
                                frame True {
                                n9292 = local read "VISA Refnum in\nfor Pump"() -> (w9726:refnum<visa-resource-name>)
                                n9293 = call "HardStopCurrentProcess (SubVI).vi"("VISA Refnum in"=w9726) -> ()  [unwired: 11 in]
                                }
                              }
                              n9294 = local read "VISA Refnum in\nfor Pump"() -> (w9724:refnum<visa-resource-name>)
                              n9295 = call "ProcessCompletionWaiter (SubVI).vi"("VISA Refnum in"=w9724) -> ()  [unwired: 11 in]
                            }
                          }
                        }
                      }
                      frame #2 {
                        n9296 = local read "No. of \ncleaning cycles"() -> (w9727:i32)
                        n9297 = for {
                          N: w9727 -> [_]
                          n9298 = stacked-sequence {
                            frame #0 {
                              # "Switch to Port-4"
                              # "Port-4 of pump is connected to Buffer-A"
                              n9299 = local read "VISA Refnum in\nfor Pump"() -> (w9730:refnum<visa-resource-name>)
                              n9300 = local write "Pause Data Collection"(TRUE ("Pause Data Collection")) -> ()
                              n9301 = call "PortChanger (SubVI).vi"("Port Number"="7", "VISA Refnum in"=w9730) -> ()  [unwired: 10 in]
                            }
                            frame #1 {
                              n9302 = local read "VISA Refnum in\nfor Pump"() -> (w9731:refnum<visa-resource-name>)
                              n9303 = call "ProcessCompletionWaiter (SubVI).vi"("VISA Refnum in"=w9731) -> ()  [unwired: 11 in]
                            }
                            frame #2 {
                              n9304 = local read "VISA Refnum in\nfor Pump"() -> (w9736:refnum<visa-resource-name>)
                              n9305 = local read "Apparent Volume\nof Syringe"() -> (w9732:dbl)
                              n9306 = local read "Volume of Syringe"() -> (w9735:dbl)
                              n9307 = call "RPickUp(SubVI).vi"("Volume to be picked up"=w9732, "Volume of Syringe"=w9735, "Resolution of PickUP"=T2."Standard Pumping", "PickUp Flow Rate (ul/min)"=150.0, "VISA Refnum in"=w9736) -> ()  [unwired: 6 in, 1 out]
                            }
                            frame #3 {
                              n9308 = local read "Stopper that ends \nthe main loops"() -> (w9737:bool)
                              n9309 = local read "VISA Refnum in\nfor Pump"() -> (w9738:refnum<visa-resource-name>)
                              n9310 = case shown="True" w9737 {
                                frame False {
                                }
                                frame True {
                                n9311 = local read "VISA Refnum in\nfor Pump"() -> (w9739:refnum<visa-resource-name>)
                                n9312 = call "HardStopCurrentProcess (SubVI).vi"("VISA Refnum in"=w9739) -> ()  [unwired: 11 in]
                                }
                              }
                              n9313 = call "ProcessCompletionWaiter (SubVI).vi"("VISA Refnum in"=w9738) -> ()  [unwired: 11 in]
                            }
                            frame #4 {
                              # "Switch to Port-1"
                              # "Port-1 of the pump is conncted to Waste"
                              n9314 = local read "VISA Refnum in\nfor Pump"() -> (w9741:refnum<visa-resource-name>)
                              n9315 = call "PortChanger (SubVI).vi"("Port Number"="1", "VISA Refnum in"=w9741) -> ()  [unwired: 10 in]
                            }
                            frame #5 {
                              n9316 = local read "Stopper that ends \nthe main loops"() -> (w9742:bool)
                              n9317 = local read "VISA Refnum in\nfor Pump"() -> (w9743:refnum<visa-resource-name>)
                              n9318 = case shown="True" w9742 {
                                frame False {
                                }
                                frame True {
                                n9319 = local read "VISA Refnum in\nfor Pump"() -> (w9744:refnum<visa-resource-name>)
                                n9320 = call "HardStopCurrentProcess (SubVI).vi"("VISA Refnum in"=w9744) -> ()  [unwired: 11 in]
                                }
                              }
                              n9321 = call "ProcessCompletionWaiter (SubVI).vi"("VISA Refnum in"=w9743) -> ()  [unwired: 11 in]
                            }
                            frame #6 {
                              n9322 = local read "VISA Refnum in\nfor Pump"() -> (w9749:refnum<visa-resource-name>)
                              n9323 = local read "Volume of Syringe"() -> (w9748:dbl)
                              n9324 = call "GoToAbsolutePosition(SubVI).vi"("Absolute Volume Position in Syringe (in ul)"=0.0 ("Volume to be Dispensed"), "Volume of Syringe"=w9748, "Resolution of Pumping"=T2."Standard Pumping" ("Resolution for Dispensing"), "Flow Rate (ul/min)"=150.0 ("Dispense Flow Rate (ul/min)"), "VISA Refnum in"=w9749) -> ()  [unwired: 6 in, 1 out]
                            }
                            frame #7 {
                              n9325 = local read "Stopper that ends \nthe main loops"() -> (w9751:bool)
                              n9326 = case shown="True" w9751 {
                                frame False {
                                }
                                frame True {
                                n9327 = local read "VISA Refnum in\nfor Pump"() -> (w9752:refnum<visa-resource-name>)
                                n9328 = call "HardStopCurrentProcess (SubVI).vi"("VISA Refnum in"=w9752) -> ()  [unwired: 11 in]
                                }
                              }
                              n9329 = local read "VISA Refnum in\nfor Pump"() -> (w9750:refnum<visa-resource-name>)
                              n9330 = call "ProcessCompletionWaiter (SubVI).vi"("VISA Refnum in"=w9750) -> ()  [unwired: 11 in]
                            }
                          }
                        }
                      }
                      frame #3 {
                        n9331 = local read "n1"() -> (w9753:dbl)
                        n9332 = for {
                          N: w9753 -> [_]
                          n9333 = stacked-sequence {
                            frame #0 {
                              # "Switch to Port-4"
                              # "Port-4 of pump is connected to Buffer-A"
                              n9334 = local read "VISA Refnum in\nfor Pump"() -> (w9756:refnum<visa-resource-name>)
                              n9335 = local write "Pause Data Collection"(TRUE ("Pause Data Collection")) -> ()
                              n9336 = call "PortChanger (SubVI).vi"("Port Number"="4", "VISA Refnum in"=w9756) -> ()  [unwired: 10 in]
                            }
                            frame #1 {
                              n9337 = local read "VISA Refnum in\nfor Pump"() -> (w9757:refnum<visa-resource-name>)
                              n9338 = call "ProcessCompletionWaiter (SubVI).vi"("VISA Refnum in"=w9757) -> ()  [unwired: 11 in]
                            }
                            frame #2 {
                              n9339 = local read "VISA Refnum in\nfor Pump"() -> (w9762:refnum<visa-resource-name>)
                              n9340 = local read "Apparent Volume\nof Syringe"() -> (w9758:dbl)
                              n9341 = local read "Volume of Syringe"() -> (w9761:dbl)
                              n9342 = call "RPickUp(SubVI).vi"("Volume to be picked up"=w9758, "Volume of Syringe"=w9761, "Resolution of PickUP"=T2."Standard Pumping", "PickUp Flow Rate (ul/min)"=150.0, "VISA Refnum in"=w9762) -> ()  [unwired: 6 in, 1 out]
                            }
                            frame #3 {
                              n9343 = local read "Stopper that ends \nthe main loops"() -> (w9763:bool)
                              n9344 = local read "VISA Refnum in\nfor Pump"() -> (w9764:refnum<visa-resource-name>)
                              n9345 = case shown="True" w9763 {
                                frame False {
                                }
                                frame True {
                                n9346 = local read "VISA Refnum in\nfor Pump"() -> (w9765:refnum<visa-resource-name>)
                                n9347 = call "HardStopCurrentProcess (SubVI).vi"("VISA Refnum in"=w9765) -> ()  [unwired: 11 in]
                                }
                              }
                              n9348 = call "ProcessCompletionWaiter (SubVI).vi"("VISA Refnum in"=w9764) -> ()  [unwired: 11 in]
                            }
                            frame #4 {
                              # "Switch to Port-1"
                              # "Port-1 of the pump is conncted to Waste"
                              n9349 = local read "VISA Refnum in\nfor Pump"() -> (w9767:refnum<visa-resource-name>)
                              n9350 = call "PortChanger (SubVI).vi"("Port Number"="2", "VISA Refnum in"=w9767) -> ()  [unwired: 10 in]
                            }
                            frame #5 {
                              n9351 = local read "Stopper that ends \nthe main loops"() -> (w9768:bool)
                              n9352 = local read "VISA Refnum in\nfor Pump"() -> (w9769:refnum<visa-resource-name>)
                              n9353 = case shown="True" w9768 {
                                frame False {
                                }
                                frame True {
                                n9354 = local read "VISA Refnum in\nfor Pump"() -> (w9770:refnum<visa-resource-name>)
                                n9355 = call "HardStopCurrentProcess (SubVI).vi"("VISA Refnum in"=w9770) -> ()  [unwired: 11 in]
                                }
                              }
                              n9356 = call "ProcessCompletionWaiter (SubVI).vi"("VISA Refnum in"=w9769) -> ()  [unwired: 11 in]
                            }
                            frame #6 {
                              n9357 = local read "Buffer-A2 Dispense\nFlow Rate (ul/min)"() -> (w9774:dbl)
                              n9358 = local read "VISA Refnum in\nfor Pump"() -> (w9778:refnum<visa-resource-name>)
                              n9359 = local read "Volume of Syringe"() -> (w9777:dbl)
                              n9360 = call "GoToAbsolutePosition(SubVI).vi"("Absolute Volume Position in Syringe (in ul)"=0.0 ("Volume to be Dispensed"), "Volume of Syringe"=w9777, "Resolution of Pumping"=T2."Standard Pumping" ("Resolution for Dispensing"), "Flow Rate (ul/min)"=w9774, "VISA Refnum in"=w9778) -> ()  [unwired: 6 in, 1 out]
                              n9361 = local write "External Valve \nOpen"(FALSE ("External Valve \nOpen")) -> ()
                              n9362 = local write "Valve V2 Open"(FALSE ("Valve V2 Open")) -> ()
                              n9363 = local write "Valve V1 Open"(TRUE ("Valve V1 Open")) -> ()
                            }
                            frame #7 {
                              n9364 = local read "Stopper that ends \nthe main loops"() -> (w9780:bool)
                              n9365 = case shown="True" w9780 {
                                frame False {
                                }
                                frame True {
                                n9366 = local read "VISA Refnum in\nfor Pump"() -> (w9781:refnum<visa-resource-name>)
                                n9367 = call "HardStopCurrentProcess (SubVI).vi"("VISA Refnum in"=w9781) -> ()  [unwired: 11 in]
                                }
                              }
                              n9368 = local read "VISA Refnum in\nfor Pump"() -> (w9779:refnum<visa-resource-name>)
                              n9369 = call "ProcessCompletionWaiter (SubVI).vi"("VISA Refnum in"=w9779) -> ()  [unwired: 11 in]
                            }
                          }
                        }
                      }
                      frame #4 {
                        n9370 = local write "Start the Process"(FALSE ("Start the Process")) -> ()
                      }
                    }
                  }
                }
              }
              frame True {
                n9371 = local write "Pause Data Collection"(FALSE ("Pause Data Collection")) -> ()
              }
            }
          }
          frame "Check_Suction_Valve_functionality" {
            n9372 = local read "Start the Process"() -> (w9784:bool)
            n9373 = case shown="True" w9784 {
              frame False {
              }
              frame True {
                n9374 = while {
                  stop <- w9787 stop-if-true
                  n9375 = local read "Suction On/Off"() -> (w9785:bool)
                  n9376 = case shown="True" w9785 {
                    frame False {
                    }
                    frame True {
                      n9377 = stacked-sequence {
                        frame #0 {
                          n9378 = while {
                            stop <- w9788 stop-if-true
                            n9379 = local read "Stop for End of \nExperiment \nand Data Writing"() -> (w9790:bool)
                            n9380 = local read "Suction Pressure\nfor EM-grid \nDeposition (mbar)"() -> (w9793:sgl)
                            n9381 = local read "Suction On/Off"() -> (w9791:bool)
                            n9382 = call <vilib>:"fgt set pressure.vi"("pressure"=w9793, "pressureIndex"=u32 1) -> ()  [unwired: 9 in, 1 out]
                            n9383 = Not(x=w9791) -> (.not. x?=w9789:bool)
                            n9384 = Or(x=w9789, y=w9790) -> (x .or. y?=w9788:bool)
                            n9385 = Wait (ms)(milliseconds to wait=u32 100) -> ()  [unwired: 1 out]
                          }
                        }
                        frame #1 {
                          n9386 = for {
                            N: 2 -> [_]
                            n9387 = while {
                              stop <- w9798 stop-if-true
                              n9388 = local read "Stop for End of \nExperiment \nand Data Writing"() -> (w9800:bool)
                              n9389 = local read "Suction On/Off"() -> (w9801:bool)
                              n9390 = call <vilib>:"fgt set pressure.vi"("pressure"=sgl 0.0, "pressureIndex"=u32 1) -> ()  [unwired: 9 in, 1 out]
                              n9391 = Not(x=w9801) -> (.not. x?=w9799:bool)
                              n9392 = Or(x=w9799, y=w9800) -> (x .or. y?=w9798:bool)
                              n9393 = Wait (ms)(milliseconds to wait=u32 100) -> ()  [unwired: 1 out]
                            }
                            n9394 = Wait (ms)(milliseconds to wait=u32 400) -> ()  [unwired: 1 out]
                          }
                        }
                      }
                    }
                  }
                  n9395 = local read "Stop for End of \nExperiment \nand Data Writing"() -> (w9787:bool)
                  n9396 = Wait (ms)(milliseconds to wait=u32 100) -> ()  [unwired: 1 out]
                }
              }
            }
          }
          frame "Automated Plunging alone using purified protein from SEC column" {
            n9397 = local read "Stopper that ends \nthe main loops"() -> (w9804:bool)
            n9398 = case shown="False" w9804 {
              frame False {
                n9399 = local read "Start the Process"() -> (w9805:bool)
                n9400 = case shown="True" w9805 {
                  frame False {
                    n9401 = local read "Stopper that ends \nthe main loops"() -> (w9807:bool)
                    n9402 = local read "Start the Process"() -> (w9806:bool)
                    n9403 = Or(x=w9807, y=w9806) -> (x .or. y?=w9808:bool)
                    n9404 = case shown="False" w9808 {
                      frame False {
                        n9405 = while {
                          stop <- w9811 stop-if-true
                          n9406 = local read "Stop for End of \nExperiment \nand Data Writing"() -> (w9810:bool)
                          n9407 = local read "Stopper that ends \nthe main loops"() -> (w9813:bool)
                          n9408 = local read "Start the Process"() -> (w9812:bool)
                          n9409 = Wait (ms)(milliseconds to wait=u32 10) -> ()  [unwired: 1 out]
                          n9410 = Or(x=w9813, y=w9812) -> (x .or. y?=w9811:bool)
                          n9411 = local write "Stopper that ends \nthe main loops"(w9810) -> ()
                        }
                        n9412 = One Button Dialog(message="Please Select the Process and Press 'Start the Process' Button") -> ()  [unwired: 1 in, 1 out]
                      }
                      frame True {
                      }
                    }
                  }
                  frame True {
                    # "Elute Column-1, Divert Sample into Column-2, Elute column-2 and Divert the sample onto Grid"
                    n9413 = stacked-sequence {
                      frame #0 {
                        # "Sets suction pressure to zeros"
                        # "Switch to Port-5/8"
                        # "Port-5/8 of pump is connected to Buffer-C1/C2"
                        n9414 = local read "VISA Refnum in\nfor Pump"() -> (w9827:refnum<visa-resource-name>)
                        n9415 = Wait (ms)(milliseconds to wait=u32 500) -> ()  [unwired: 1 out]
                        n9416 = local write "Pause Data Collection"(TRUE ("Pause Data Collection")) -> ()
                        n9417 = local read "Port for \nC2-Elution"() -> (w9822:string)
                        n9418 = call "PortChanger (SubVI).vi"("Port Number"=w9822, "VISA Refnum in"=w9827) -> ()  [unwired: 10 in]
                        n9419 = local write "Valve V1 Open"(FALSE ("Valve V1 Open")) -> ()
                        n9420 = local write "Valve V2 Open"(FALSE ("Valve V2 Open")) -> ()
                        n9421 = local write "Valve V3 Open"(FALSE ("Valve V3 Open")) -> ()
                        n9422 = local write "Valve V4 Open"(FALSE ("Valve V4 Open")) -> ()
                        n9423 = local write "External Valve \nOpen"(FALSE ("External Valve \nOpen")) -> ()
                        n9424 = local write "Valve V8 Open"(FALSE ("Valve V8 Open")) -> ()
                        n9425 = local write "Valve V5 Open"(FALSE ("Valve V5 Open")) -> ()
                        n9426 = local write "Valve V6 Open"(FALSE ("Valve V6 Open")) -> ()
                        n9427 = local write "Valve V7 Open"(FALSE ("Valve V7 Open")) -> ()
                        n9428 = call <vilib>:"fgt set pressure.vi"("pressure"=sgl 0.0, "pressureIndex"=u32 1) -> ()  [unwired: 9 in, 1 out]
                      }
                      frame #1 {
                        n9429 = local read "VISA Refnum in\nfor Pump"() -> (w9831:refnum<visa-resource-name>)
                        n9430 = call "ProcessCompletionWaiter (SubVI).vi"("VISA Refnum in"=w9831) -> ()  [unwired: 11 in]
                        n9431 = local write "Start the Process"(FALSE ("Start the Process")) -> ()
                      }
                      frame #2 {
                        n9432 = local write "Elution of Column-1"(FALSE ("Elution of Column-1")) -> ()
                        n9433 = local write "Volume being Injected \nin this process"(0.0 ("Volume being Injected \nin this process")) -> ()
                        n9434 = local write "Elution of Column-2"(TRUE ("Elution of Column-2")) -> ()
                      }
                      frame #3 {
                        # "If Yes, it will clean the SEC buffer from port-8 tubing else it will clean the pump valve a bit"
                        n9435 = local read "Clean the \nBuffer-C2 tubing"() -> (w9835:bool)
                        n9436 = case shown="False" w9835 {
                          frame False {
                            n9437 = stacked-sequence {
                              frame #0 {
                                n9438 = local read "VISA Refnum in\nfor Pump"() -> (w9837:refnum<visa-resource-name>)
                                n9439 = local read "Port for \nC2-Elution"() -> (w9836:string)
                                n9440 = call "PortChanger (SubVI).vi"("Port Number"=w9836, "VISA Refnum in"=w9837) -> ()  [unwired: 10 in]
                              }
                              frame #1 {
                                n9441 = local read "VISA Refnum in\nfor Pump"() -> (w9838:refnum<visa-resource-name>)
                                n9442 = call "ProcessCompletionWaiter (SubVI).vi"("VISA Refnum in"=w9838) -> ()  [unwired: 11 in]
                              }
                              frame #2 {
                                n9443 = local read "Buffer-C2 Pumping\nResolution"() -> (w9841:T2)
                                n9444 = local read "VISA Refnum in\nfor Pump"() -> (w9843:refnum<visa-resource-name>)
                                n9445 = local read "V-S"() -> (w9839:dbl)
                                n9446 = local read "Volume of Syringe"() -> (w9842:dbl)
                                n9447 = call "RPickUp(SubVI).vi"("Volume to be picked up"=w9839, "Volume of Syringe"=w9842, "Resolution of PickUP"=w9841, "PickUp Flow Rate (ul/min)"=150.0, "VISA Refnum in"=w9843) -> ()  [unwired: 6 in, 1 out]
                              }
                              frame #3 {
                                n9448 = local read "Stopper that ends \nthe main loops"() -> (w9844:bool)
                                n9449 = local read "VISA Refnum in\nfor Pump"() -> (w9845:refnum<visa-resource-name>)
                                n9450 = case shown="True" w9844 {
                                frame False {
                                }
                                frame True {
                                n9451 = local read "VISA Refnum in\nfor Pump"() -> (w9846:refnum<visa-resource-name>)
                                n9452 = call "HardStopCurrentProcess (SubVI).vi"("VISA Refnum in"=w9846) -> ()  [unwired: 11 in]
                                }
                                }
                                n9453 = call "ProcessCompletionWaiter (SubVI).vi"("VISA Refnum in"=w9845) -> ()  [unwired: 11 in]
                              }
                              frame #4 {
                                n9454 = local read "VISA Refnum in\nfor Pump"() -> (w9848:refnum<visa-resource-name>)
                                n9455 = call "PortChanger (SubVI).vi"("Port Number"="1", "VISA Refnum in"=w9848) -> ()  [unwired: 10 in]
                              }
                              frame #5 {
                                n9456 = local read "Stopper that ends \nthe main loops"() -> (w9849:bool)
                                n9457 = local read "VISA Refnum in\nfor Pump"() -> (w9850:refnum<visa-resource-name>)
                                n9458 = case shown="True" w9849 {
                                frame False {
                                }
                                frame True {
                                n9459 = local read "VISA Refnum in\nfor Pump"() -> (w9851:refnum<visa-resource-name>)
                                n9460 = call "HardStopCurrentProcess (SubVI).vi"("VISA Refnum in"=w9851) -> ()  [unwired: 11 in]
                                }
                                }
                                n9461 = call "ProcessCompletionWaiter (SubVI).vi"("VISA Refnum in"=w9850) -> ()  [unwired: 11 in]
                              }
                              frame #6 {
                                n9462 = local read "VISA Refnum in\nfor Pump"() -> (w9856:refnum<visa-resource-name>)
                                n9463 = local read "Volume of Syringe"() -> (w9853:dbl)
                                n9464 = call "GoToAbsolutePosition(SubVI).vi"("Absolute Volume Position in Syringe (in ul)"=0.0, "Volume of Syringe"=w9853, "Resolution of Pumping"=T2."Standard Pumping", "Flow Rate (ul/min)"=150.0, "VISA Refnum in"=w9856) -> ()  [unwired: 6 in, 1 out]
                              }
                              frame #7 {
                                n9465 = local read "Stopper that ends \nthe main loops"() -> (w9857:bool)
                                n9466 = local read "VISA Refnum in\nfor Pump"() -> (w9858:refnum<visa-resource-name>)
                                n9467 = case shown="True" w9857 {
                                frame False {
                                }
                                frame True {
                                n9468 = local read "VISA Refnum in\nfor Pump"() -> (w9859:refnum<visa-resource-name>)
                                n9469 = call "HardStopCurrentProcess (SubVI).vi"("VISA Refnum in"=w9859) -> ()  [unwired: 11 in]
                                }
                                }
                                n9470 = call "ProcessCompletionWaiter (SubVI).vi"("VISA Refnum in"=w9858) -> ()  [unwired: 11 in]
                              }
                            }
                          }
                          frame True {
                            n9471 = for {
                              N: 2 -> [_]
                              n9472 = stacked-sequence {
                                frame #0 {
                                n9473 = local read "VISA Refnum in\nfor Pump"() -> (w9862:refnum<visa-resource-name>)
                                n9474 = local read "Port for \nC2-Elution"() -> (w9861:string)
                                n9475 = call "PortChanger (SubVI).vi"("Port Number"=w9861, "VISA Refnum in"=w9862) -> ()  [unwired: 10 in]
                                }
                                frame #1 {
                                n9476 = local read "VISA Refnum in\nfor Pump"() -> (w9863:refnum<visa-resource-name>)
                                n9477 = call "ProcessCompletionWaiter (SubVI).vi"("VISA Refnum in"=w9863) -> ()  [unwired: 11 in]
                                }
                                frame #2 {
                                n9478 = local read "Buffer-C2 Pumping\nResolution"() -> (w9866:T2)
                                n9479 = local read "VISA Refnum in\nfor Pump"() -> (w9868:refnum<visa-resource-name>)
                                n9480 = local read "Apparent Volume\nof Syringe"() -> (w9864:dbl)
                                n9481 = local read "Volume of Syringe"() -> (w9867:dbl)
                                n9482 = call "RPickUp(SubVI).vi"("Volume to be picked up"=w9864, "Volume of Syringe"=w9867, "Resolution of PickUP"=w9866, "PickUp Flow Rate (ul/min)"=150.0, "VISA Refnum in"=w9868) -> ()  [unwired: 6 in, 1 out]
                                }
                                frame #3 {
                                n9483 = local read "Stopper that ends \nthe main loops"() -> (w9869:bool)
                                n9484 = local read "VISA Refnum in\nfor Pump"() -> (w9870:refnum<visa-resource-name>)
                                n9485 = case shown="True" w9869 {
                                frame False {
                                }
                                frame True {
                                n9486 = local read "VISA Refnum in\nfor Pump"() -> (w9871:refnum<visa-resource-name>)
                                n9487 = call "HardStopCurrentProcess (SubVI).vi"("VISA Refnum in"=w9871) -> ()  [unwired: 11 in]
                                }
                                }
                                n9488 = call "ProcessCompletionWaiter (SubVI).vi"("VISA Refnum in"=w9870) -> ()  [unwired: 11 in]
                                }
                                frame #4 {
                                n9489 = local read "VISA Refnum in\nfor Pump"() -> (w9873:refnum<visa-resource-name>)
                                n9490 = call "PortChanger (SubVI).vi"("Port Number"="1", "VISA Refnum in"=w9873) -> ()  [unwired: 10 in]
                                }
                                frame #5 {
                                n9491 = local read "Stopper that ends \nthe main loops"() -> (w9874:bool)
                                n9492 = local read "VISA Refnum in\nfor Pump"() -> (w9875:refnum<visa-resource-name>)
                                n9493 = case shown="True" w9874 {
                                frame False {
                                }
